vi "SetList SWI to Devices.vi"(8 "error in (no error)":errorcluster, 9 "SWI table":string[][](array[string]), 10 "DevNums In":i32[](array[numeric]), 11 "Devices queue":refnum<queue>) -> (0 "error out":errorcluster, 2 "Devices out":refnum<class "Device.lvclass">[](array[class]), 3 "Devices queue out":refnum<queue>)   [LabVIEW 2013]
doc: "Loop over devices and write corresponding portion of SetList SWI (table) to each device. (Data only, not appearance in table!)"
uses:
  Device/Device.lvclass
panel:
  # "Want to update SetList SWI (data) changes to devices!"
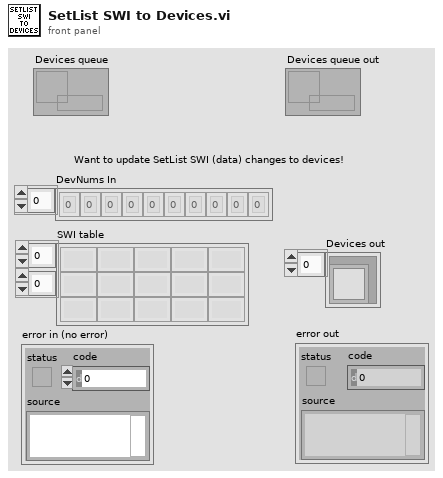
[diagram p1: front panel]
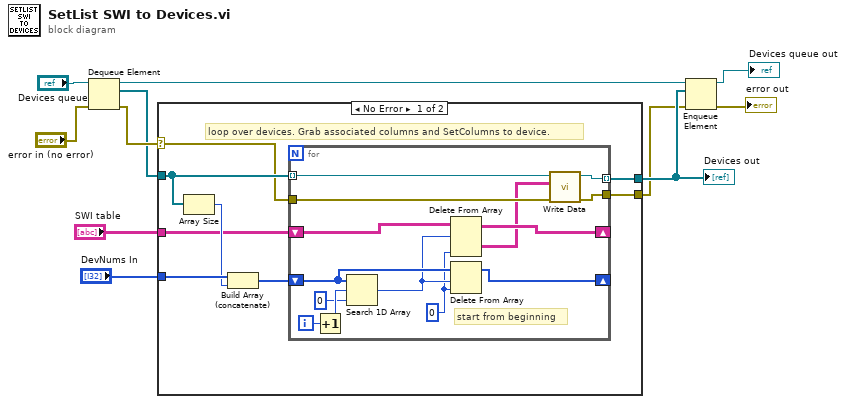
[diagram p0: block diagram]
diagram:
  n1 = Dequeue Element(queue="Devices queue", error in (no error)="error in (no error)") -> (queue out=w5:refnum<queue>, element=w6:refnum<class "Device.lvclass">[], error out=w7:errorcluster)  [unwired: 1 in, 1 out]
  n2 = case shown="No Error" w7 {
    selector: w7 -> [w12 w35]
    tunnel: [w19 w34] -> w4
    tunnel: w6 -> [w18 w34]
    tunnel: "DevNums In" -> [w17 _]
    tunnel: "SWI table" -> [w14 _]
    tunnel: [w13 w35] -> w3
    frame No Error {
      # "loop over devices. Grab associated columns and SetColumns to device."
      n3 = Array Size(array=w18) -> (size(s)=w15:i32)
      n4 = Build Array (concatenate)(w17, w15) -> (w16:i32[])
      n5 = for {
        tunnel: w18 -> [w33] mode=indexing
        tunnel: [w32] -> w19 mode=indexing
        shift-right: [w28] -> _
        shift-left: w14 -> [w29]
        shift-right: [w26] -> _
        shift-left: w16 -> [w27]
        tunnel: [w23] -> w13
        tunnel: w12 -> [w22]
        i -> [w31]
        w20 = 0 ("start index (0)")
        # "start from beginning"
        n6 = Increment(x=w31) -> (x+1=w30:i32)
        n7 = Search 1D Array(1D array=w27, element=w30, start index (0)=0) -> (index of element=w24:i32)
        n8 = Delete From Array(array=w29, length=w24, index (col)=w20) -> (deleted portion=w21:string[][], array with subset deleted=w28:string[][])  [unwired: 1 in]
        n9 = Delete From Array(array=w27, length=w24, index=w20) -> (array with subset deleted=w26:i32[])  [unwired: 1 out]
        n10 = call-dynamic "Write Data.vi"("error in (no error)"=w22, "Data"=w21, "Device in"=w33) -> ("error out"=w23:errorcluster, "Device Out"=w32:refnum<class "Device.lvclass">)  [unwired: 7 in]
      }
    }
    frame Error {
    }
  }
  "Devices out" <- w4
  n11 = Enqueue Element(queue=w5, element=w4, error in (no error)=w3) -> (queue out=→"Devices queue out":refnum<queue>, error out=→"error out":errorcluster)  [unwired: 1 in, 1 out]
